vi "Module Loop.vi"(8 "error in (no error)":errorcluster, 11 "GenericGuiAO in":refnum<class "GenericGuiAO.lvclass">) -> (0 "error out":errorcluster, 3 "GenericGuiAO out":refnum<class "GenericGuiAO.lvclass">)   [LabVIEW 2020, in "VolatusDAQGenericGUI.lvlib" / "GenericGuiAO.lvclass"]
uses:
  GenericGuiAO.lvclass
  C:/dev/lv20CE/relink/lv-volatus/Volatus/Module/Module.lvclass
  Volatus/Module/Module.lvclass/Module.ctl
  Volatus/MessageQ/MessageQ.lvclass/MessageQ.ctl
  GenericGuiAO.lvclass/GenericGuiAO.ctl
  Volatus/Module/Module.lvclass
  <vilib>/Utility/error.llb/Error Cluster From Error Code.vi
  Volatus/MessageQ/MessageQ.lvclass
  VolatusDAQGenericGUI.lvlib
  C:/dev/lv20CE/relink/lv-volatus/VolatusDAQGenericGUI/GenericGuiAO/GenericGuiAO.lvclass
  Volatus/VolatusAPI/VolatusAPI.lvclass
  VolatusGUI/GUI Helper/GUI Helper.lvclass
panel:
  in  "Tree":string(tree)
  out "Cover":string="\n\n\n\n\n\n\nSelect Channel to command"
  in  "Numeric":dbl
  out "Channel":string
  in  "Send Command":bool
  in  "Live Command":bool
  in  "Slide":dbl(slide) scale=0.0..10.0
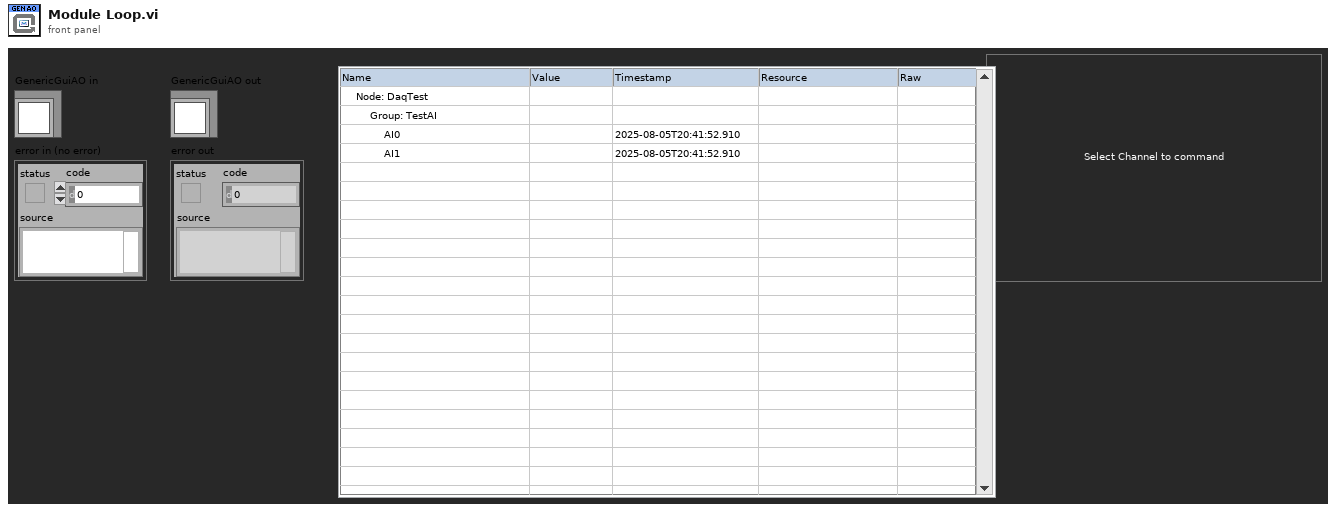
[diagram p1: front panel]
types:
  T1 = enum32{"Invalid", "Standard", "Closed", "Hidden", "Minimized", "Maximized"}
  T2 = typedef "VolatusDAQGenericGUI.lvlib/Group Info.ctl" = cluster{"Group":refnum<class "Group.lvclass">, "Channel Names":string[], "Resources":string[], "Node":string, "Task":string}
  T3 = enum8{"Enabled", "Disabled", "Disabled and Grayed Out"}
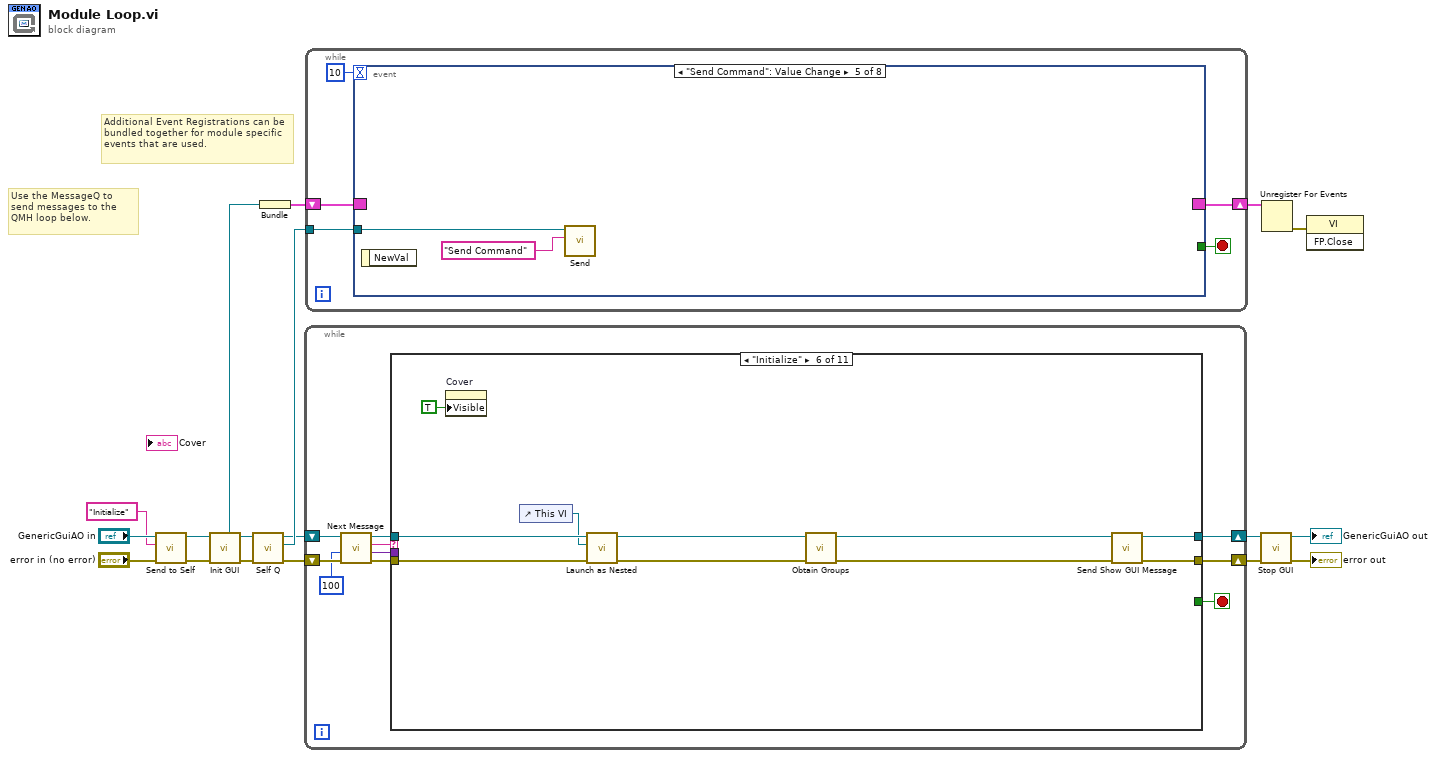
[diagram p0: block diagram]
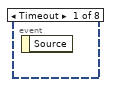
[diagram p2: hidden frame]
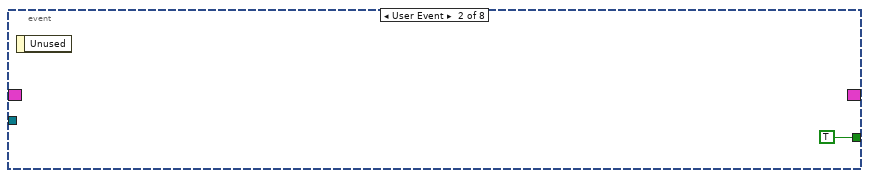
[diagram p3: hidden frame]
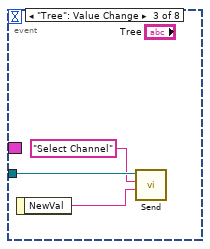
[diagram p4: hidden frame]
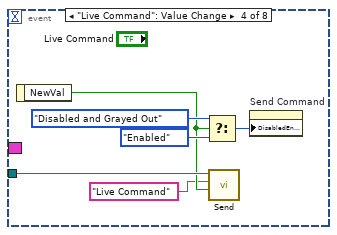
[diagram p5: hidden frame]
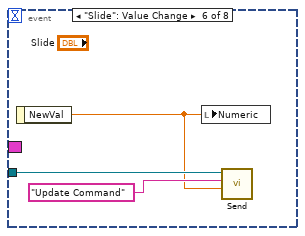
[diagram p6: hidden frame]
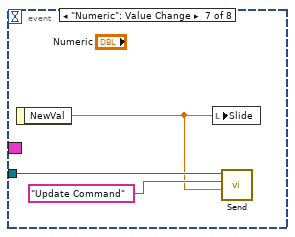
[diagram p7: hidden frame]
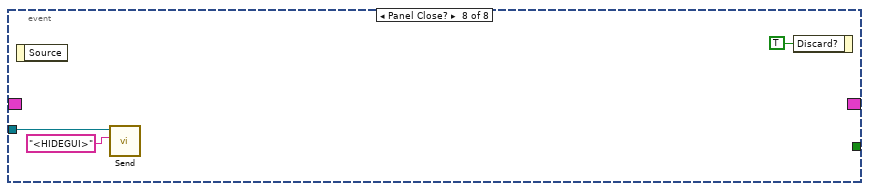
[diagram p8: hidden frame]
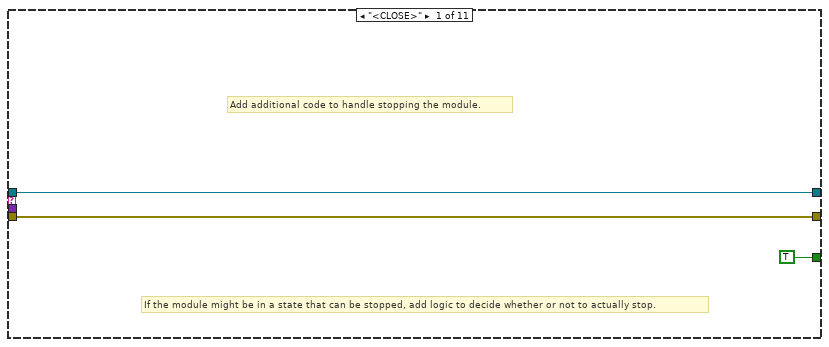
[diagram p9: hidden frame]
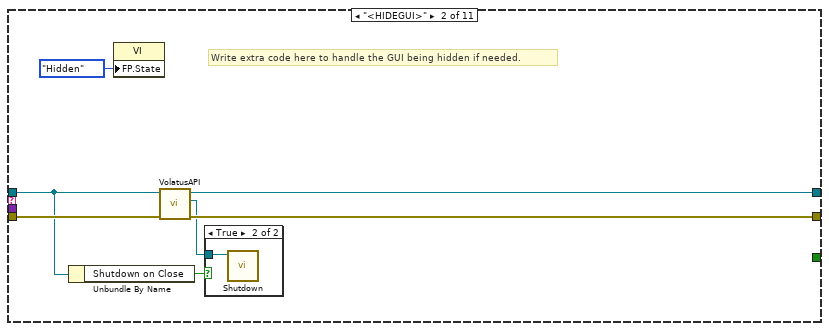
[diagram p10: hidden frame]
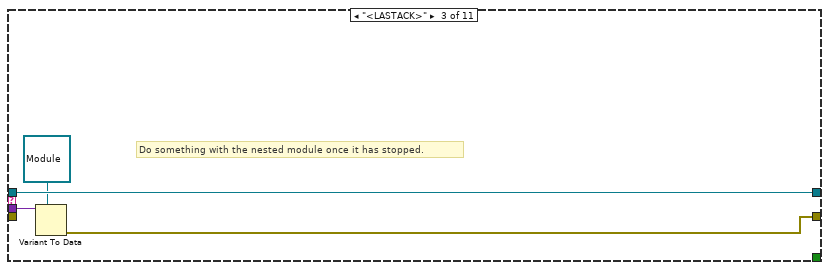
[diagram p12: hidden frame]
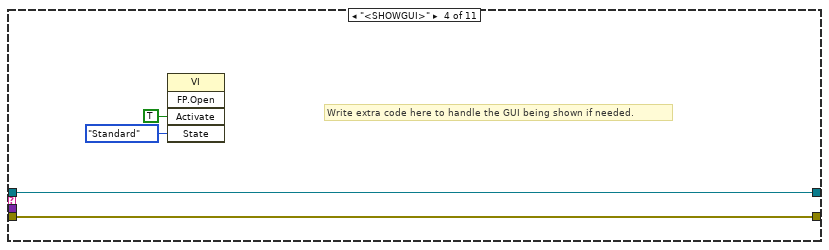
[diagram p13: hidden frame]
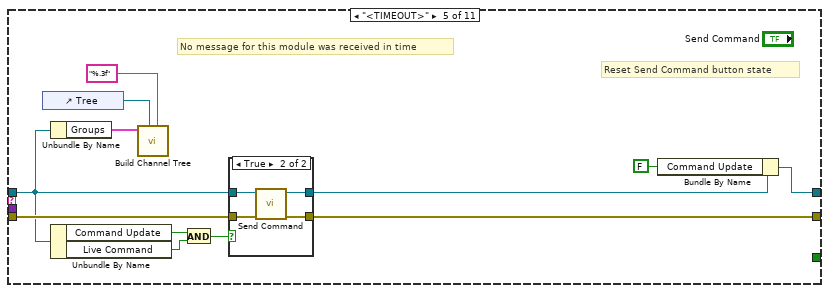
[diagram p14: hidden frame]
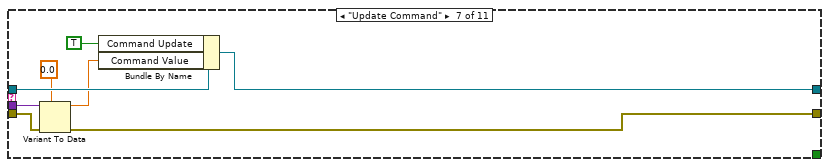
[diagram p16: hidden frame]
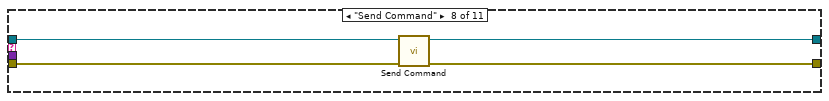
[diagram p17: hidden frame]
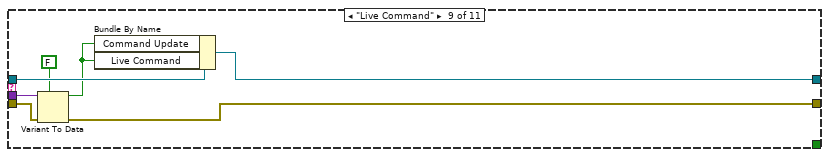
[diagram p18: hidden frame]
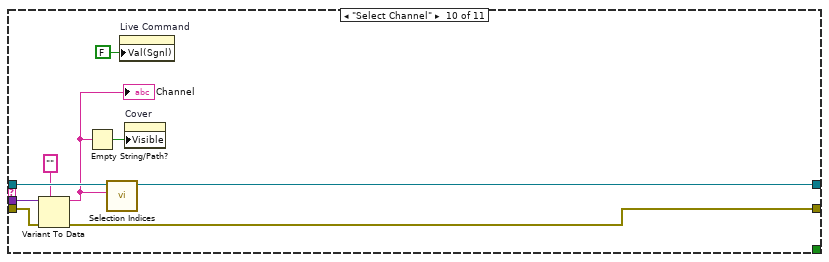
[diagram p19: hidden frame]
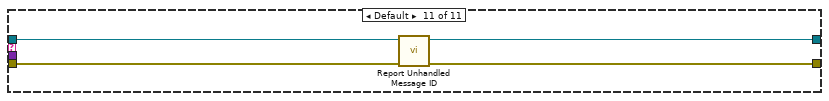
[diagram p20: hidden frame]
diagram:
  # "Additional Event Registrations can be bundled together for module specific events that are used."
  # "Use the MessageQ to send messages to the QMH loop below."
  n1 = call "Send to Self.vi"("error in (no error)"="error in (no error)", "Message ID"="Initialize", "Module in"="GenericGuiAO in") -> ("error out"=w6:errorcluster, "Module out"=w4:refnum<class "GenericGuiAO.lvclass">)  [unwired: 7 in]
  n2 = call "Init GUI.vi"("Module in"=w4) -> ("Module out"=w10:refnum<class "GenericGuiAO.lvclass">, "Event Reg"=w15:refnum<event-registration>)  [unwired: 9 in]
  n3 = call "Self Q.vi"("Module in"=w10) -> ("Self Q"=w9:refnum<class "MessageQ.lvclass">, "Module out"=w8:refnum<class "GenericGuiAO.lvclass">)  [unwired: 9 in]
  n4 = Bundle("Event Reg"=w15) -> (w11:cluster{"Event Reg":refnum<event-registration>})  [unwired: 1 in]
  n5 = while {
    shift-right: [w21] -> w13
    shift-left: w8 -> [w26]
    shift-right: [w20] -> w14
    shift-left: w6 -> [w25]
    stop <- w19 stop-if-true
    n6 = call "Next Message.vi"("error in (no error)"=w25, "Timeout ms (-1)"=100, "Module in"=w26) -> ("error out"=w24:errorcluster, "Data"=w18:variant, "ID"=w23:string, "Module out"=w22:refnum<class "GenericGuiAO.lvclass">)  [unwired: 5 in]
    n7 = case shown="\"Initialize\"" w23 {
      tunnel: w24 -> [w27 w35 _ w43 w56 w72 w79 w84 w90 w99 w104]
      tunnel: w22 -> [w28 w30 w40 w44 w48 w65 w80 w82 w91 w100 w102]
      tunnel: [w28 w31 w40 w44 w53 w68 w75 w81 w86 w93 w101] -> w21
      tunnel: [w27 w35 w37 w43 w49 w70 w78 w83 w89 w98 w103] -> w20
      tunnel: [TRUE _ _ _ _ _ _ _ _ _ _] -> w19
      tunnel: w18 -> [_ _ w39 _ _ _ w77 _ w88 w97 _]
      frame "<CLOSE>" {
        # "If the module might be in a state that can be stopped, add logic to decide whether or not to actually stop."
        # "Add additional code to handle stopping the module."
      }
      frame "<HIDEGUI>" {
        # "Write extra code here to handle the GUI being hidden if needed."
        n8 = Unbundle By Name(w30) -> ("Shutdown on Close"=w33:bool)
        n9 = property class="VI"("FP.State"=T1."Hidden" ("Front Panel Window:State")) -> ()  [unwired: 2 in, 2 out]
        n10 = call "VolatusAPI.vi"("Module in"=w30) -> ("VolatusAPI"=w32:refnum<class "VolatusAPI.lvclass">, "Module out"=w31:refnum<class "GenericGuiAO.lvclass">)  [unwired: 9 in]
        n11 = case shown="True" w33 {
          tunnel: w32 -> [_ w36]
          frame False {
          }
          frame True {
            n12 = call "Shutdown.vi"("VolatusAPI in"=w36) -> ()  [unwired: 9 in, 2 out]
          }
        }
      }
      frame "<LASTACK>" {
        # "Do something with the nested module once it has stopped."
        n13 = Variant To Data(type=refnum<class "Module.lvclass"> refnum ("Volatus:Module"), Variant=w39) -> (error out=w37:errorcluster)  [unwired: 1 in, 1 out]
      }
      frame "<SHOWGUI>" {
        # "Write extra code here to handle the GUI being shown if needed."
        n14 = invoke class="VI" method="FP.Open"("Activate"=TRUE ("Activate?"), "State"=T1."Standard") -> ()  [unwired: 3 in, 5 out]
      }
      frame "<TIMEOUT>" {
        # "Reset Send Command button state"
        # "No message for this module was received in time"
        n15 = control-ref of="Tree"() -> (w54:refnum<vi>)
        n16 = Unbundle By Name(w48) -> ("Groups"=w55:T2[])
        n17 = Unbundle By Name(w48) -> ("Command Update"=w51:bool, "Live Command"=w50:bool)
        n18 = call "Build Channel Tree.vi"("Value Format"="%.3f", "Tree"=w54, "Groups"=w55) -> ()  [unwired: 9 in]
        n19 = And(x=w51, y=w50) -> (x .and. y?=w46:bool)
        n20 = case shown="True" w46 {
          tunnel: w56 -> [w57 w62]
          tunnel: [w57 w61] -> w49
          tunnel: w48 -> [w58 w60]
          tunnel: [w58 w59] -> w47
          frame False {
          }
          frame True {
            n21 = call "Send Command.vi"("error in (no error)"=w62, "GenericGuiAO in"=w60) -> ("error out"=w61:errorcluster, "GenericGuiAO out"=w59:refnum<class "GenericGuiAO.lvclass">)  [unwired: 8 in]
          }
        }
        n22 = Bundle By Name(cluster=w47, "Command Update"=FALSE) -> (w53:refnum<class "GenericGuiAO.lvclass">)
      }
      frame "Initialize" {
        n23 = property on="Cover" class="Str"("Visible"=TRUE) -> ()  [unwired: 2 in, 2 out]
        n24 = control-ref of="This VI"() -> (w63:refnum<vi>)
        n25 = call "Launch as Nested.vi"("error in (no error)"=w72, "GUI"=w63, "Parent in"=w65) -> ("error out"=w66:errorcluster, "Parent"=w64:refnum<class "GenericGuiAO.lvclass">)  [unwired: 6 in, 1 out]
        n26 = call "Obtain Groups.vi"("error in (no error)"=w66, "GenericGuiAO in"=w64) -> ("error out"=w71:errorcluster, "GenericGuiAO out"=w69:refnum<class "GenericGuiAO.lvclass">)  [unwired: 8 in]
        n27 = call "Send Show GUI Message.vi"("error in (no error)"=w71, "Module in"=w69) -> ("error out"=w70:errorcluster, "Module out"=w68:refnum<class "GenericGuiAO.lvclass">)  [unwired: 8 in]
      }
      frame "Update Command" {
        n28 = Variant To Data(error in=w79, type=0.0, Variant=w77) -> (data=w74:dbl, error out=w78:errorcluster)
        n29 = Bundle By Name(cluster=w80, "Command Update"=TRUE, "Command Value"=w74) -> (w75:refnum<class "GenericGuiAO.lvclass">)
      }
      frame "Send Command" {
        n30 = call "Send Command.vi"("error in (no error)"=w84, "GenericGuiAO in"=w82) -> ("error out"=w83:errorcluster, "GenericGuiAO out"=w81:refnum<class "GenericGuiAO.lvclass">)  [unwired: 8 in]
      }
      frame "Live Command" {
        n31 = Variant To Data(error in=w90, type=FALSE, Variant=w88) -> (data=w85:bool, error out=w89:errorcluster)
        n32 = Bundle By Name(cluster=w91, "Command Update"=w85, "Live Command"=w85) -> (w86:refnum<class "GenericGuiAO.lvclass">)
      }
      frame "Select Channel" {
        n33 = Variant To Data(error in=w99, type="", Variant=w97) -> (data=w92:string, error out=w98:errorcluster)
        "Channel" <- w92
        n34 = Empty String/Path?(string/path=w92) -> (empty?=w95:bool)
        n35 = call "Selection Indices.vi"("Channel Tree Tag"=w92, "GenericGuiAO in"=w100) -> ("GenericGuiAO out"=w93:refnum<class "GenericGuiAO.lvclass">)  [unwired: 8 in, 1 out]
        n36 = property on="Live Command" class="Bool (strict)"("Val(Sgnl)"=FALSE ("Value (Signaling)")) -> ()  [unwired: 2 in, 2 out]
        n37 = property on="Cover" class="Str"("Visible"=w95) -> ()  [unwired: 2 in, 2 out]
      }
      frame Default {
        n38 = call "Report Unhandled Message ID.vi"("error in (no error)"=w104, "Module in"=w102) -> ("error out"=w103:errorcluster, "Module out"=w101:refnum<class "GenericGuiAO.lvclass">)  [unwired: 8 in]
      }
    }
  }
  n39 = while {
    tunnel: w9 -> [w109]
    shift-right: [w107] -> w12
    shift-left: w11 -> [w108]
    stop <- w106 stop-if-true
    n40 = event shown="[4] \"Send Command\": Value Change" {
      selector: w108 -> [_ _ _ _ _ _ _ _]
      dyn-events: [_ _ _ _ _ _ _ _] -> w107
      timeout: 10 -> [_ _ _ _ _ _ _ _]
      tunnel: w109 -> [_ _ w113 w116 w121 w124 w127 w129]
      tunnel: [_ TRUE _ _ _ _ _ _] -> w106
      event Timeout {
        n41 = event-data() -> ()  [unwired: 1 in, 1 out]
      }
      event User Event {
        n42 = event-data() -> ()  [unwired: 1 in, 1 out]
      }
      event "Tree": Value Change {
        n43 = event-data() -> ("NewVal"=w112:string)  [unwired: 1 in]
        n44 = call "Send.vi"("Data"=w112, "ID"="Select Channel", "MessageQ in"=w113) -> ()  [unwired: 7 in, 2 out]
      }
      event "Live Command": Value Change {
        n45 = event-data() -> ("NewVal"=w115:bool)  [unwired: 1 in]
        n46 = Select(t=T3."Disabled and Grayed Out" ("Disabled"), s=w115, f=T3."Enabled" ("Disabled")) -> (s? t:f=w117:T3)
        n47 = call "Send.vi"("Data"=w115, "ID"="Live Command", "MessageQ in"=w116) -> ()  [unwired: 7 in, 2 out]
        n48 = property on="Send Command" class="Bool"("DisabledEnum"=w117) -> ()  [unwired: 2 in, 2 out]
      }
      event "Send Command": Value Change {
        n49 = event-data() -> ()  [unwired: 1 in, 1 out]
        n50 = call "Send.vi"("ID"="Send Command", "MessageQ in"=w121) -> ()  [unwired: 8 in, 2 out]
      }
      event "Slide": Value Change {
        n51 = event-data() -> ("NewVal"=w122:dbl)  [unwired: 1 in]
        n52 = local write "Numeric"(w122) -> ()
        n53 = call "Send.vi"("Data"=w122, "ID"="Update Command", "MessageQ in"=w124) -> ()  [unwired: 7 in, 2 out]
      }
      event "Numeric": Value Change {
        n54 = event-data() -> ("NewVal"=w125:dbl)  [unwired: 1 in]
        n55 = local write "Slide"(w125) -> ()
        n56 = call "Send.vi"("Data"=w125, "ID"="Update Command", "MessageQ in"=w127) -> ()  [unwired: 7 in, 2 out]
      }
      event Panel Close? {
        n57 = event-data() -> ()  [unwired: 1 in, 1 out]
        n58 = call "Send.vi"("ID"="<HIDEGUI>", "MessageQ in"=w129) -> ()  [unwired: 8 in, 2 out]
        n59 = event-data("Discard?"=TRUE) -> ()  [unwired: 1 in, 1 out]
      }
    }
  }
  n60 = call "Stop GUI.vi"("error in (no error)"=w14, "Module in"=w13) -> ("error out"=→"error out":errorcluster, "Module out"=→"GenericGuiAO out":refnum<class "GenericGuiAO.lvclass">)  [unwired: 8 in]
  n61 = Unregister For Events(event registration refnum=w12) -> (error out=w16:errorcluster)  [unwired: 1 in]
  n62 = invoke class="VI" method="FP.Close"(error in=w16) -> ()  [unwired: 2 in, 3 out]
